vi "Log Error.vi"(8 "error in (no error)":errorcluster, 10 "Error Data":T1, 11 "Elevator Controller Actor in":refnum<class "Elevator Controller Actor.lvclass">) -> (0 "error out":errorcluster, 3 "Elevator Controller Actor out":refnum<class "Elevator Controller Actor.lvclass">)   [LabVIEW 2019, in "Elevator Controller Actor.lvlib" / "Elevator Controller Actor.lvclass"]
uses:
  Elevator Controller Actor.lvclass
  Error Level -Enum.ctl
  Error Data.ctl
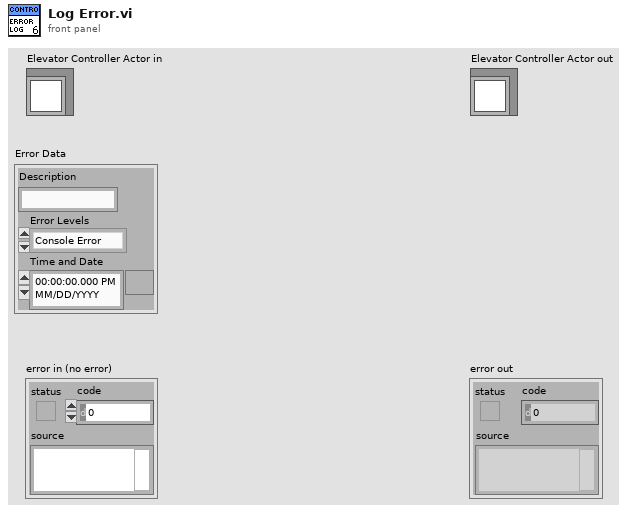
[diagram p1: front panel]
types:
  T1 = typedef "Elevator Controller Actor.lvlib/Elevator Controller Actor.lvclass/Error Data.ctl" = cluster{"Description":string, "Error Levels":T2, "Time and Date":timestamp}
  T2 = typedef "Elevator Controller Actor.lvlib/Elevator Controller Actor.lvclass/Error Level -Enum.ctl" = enum16{"Console Error", "Sensor Interface IO Error", "Process Step Error"}
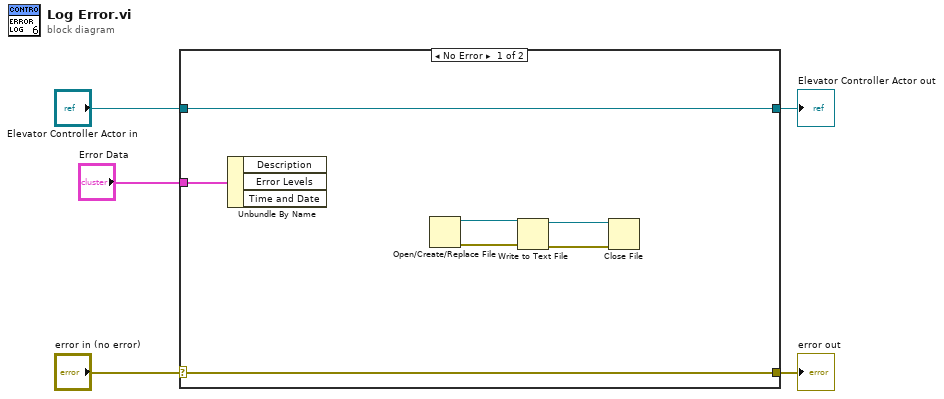
[diagram p0: block diagram]
diagram:
  n1 = case shown="No Error" "error in (no error)" {
    selector: "error in (no error)" -> [w11 w14]
    tunnel: [w11 w14] -> w4
    tunnel: [w12 w13] -> w2
    tunnel: "Elevator Controller Actor in" -> [w12 w13]
    tunnel: "Error Data" -> [w10 _]
    frame No Error {
      n2 = Unbundle By Name(w10) -> ()  [unwired: 3 out]
      n3 = Open/Create/Replace File() -> (refnum out=w9:refnum<file>, error out=w7:errorcluster)  [unwired: 6 in, 1 out]
      n4 = Write to Text File(file (use dialog)=w9, error in=w7) -> (refnum out=w8:refnum<file>, error out=w6:errorcluster)  [unwired: 2 in, 1 out]
      n5 = Close File(refnum=w8, error in=w6) -> ()  [unwired: 2 out]
    }
    frame Error {
    }
  }
  "error out" <- w4
  "Elevator Controller Actor out" <- w2
